vi "Counter with Button.vi"() -> ()   [LabVIEW 2022 SP3]
panel:
  in  "Sifirla":bool
  out "Say. Mavi":i32
  out "Say. Yesil":i32
  out "Say. Kirmizi":i32
  in  "stop":bool
  in  "Mavi":bool
  in  "Yesil":bool
  in  "Kirmizi":bool
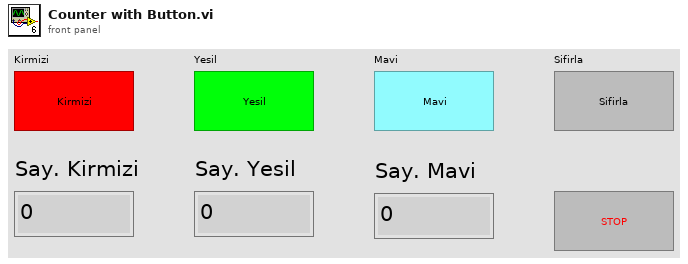
[diagram p1: front panel]
types:
  T1 = cluster{"Counters":cluster{"Say. Kirmizi":i32, "Say. Yesil":i32, "Say. Mavi":i32}}
  T2 = cluster{"Say. Kirmizi":i32, "Say. Yesil":i32, "Say. Mavi":i32}
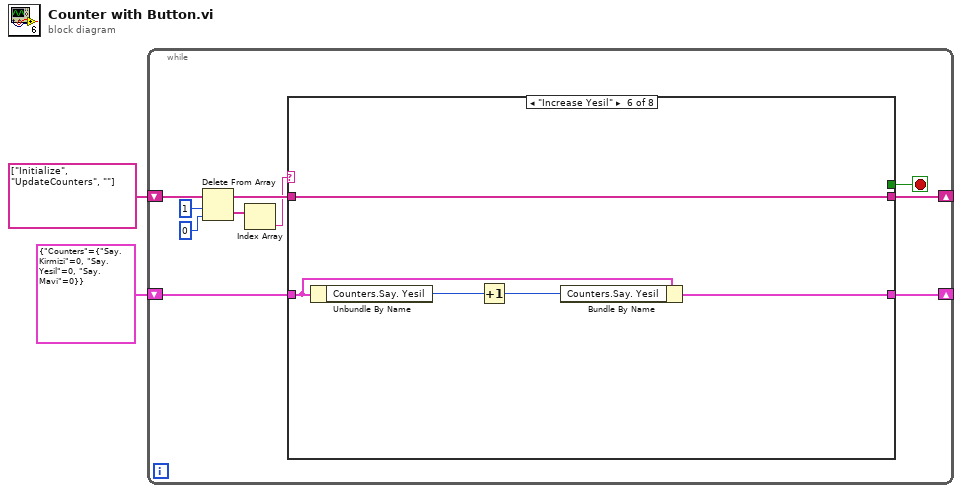
[diagram p0: block diagram]
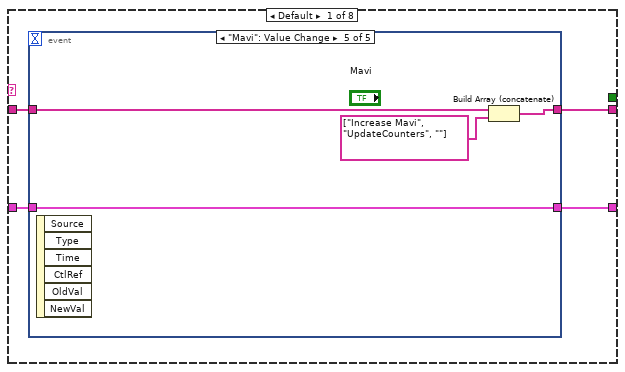
[diagram p2: hidden frame]
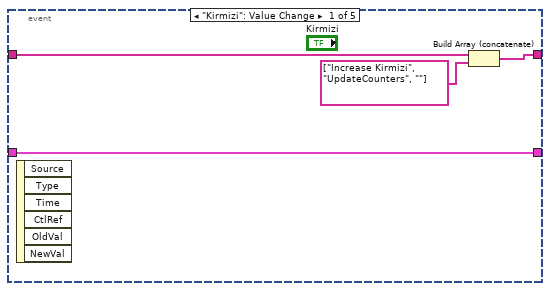
[diagram p3: hidden frame]
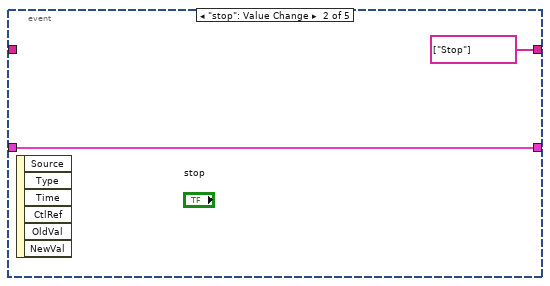
[diagram p4: hidden frame]
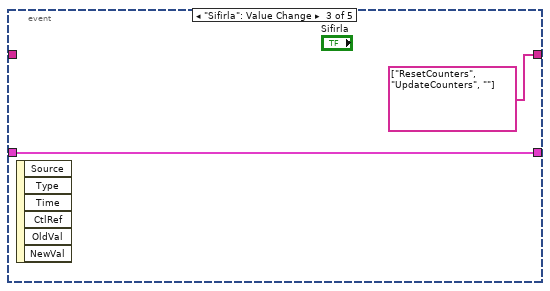
[diagram p5: hidden frame]
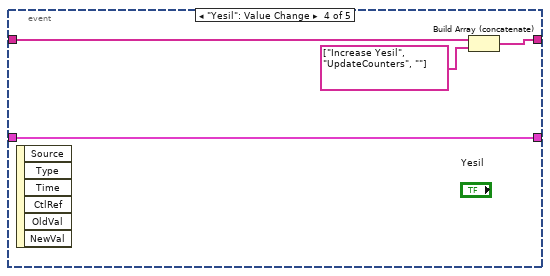
[diagram p6: hidden frame]
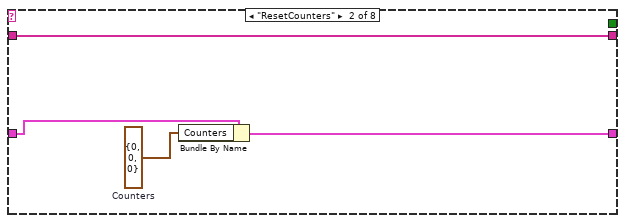
[diagram p7: hidden frame]
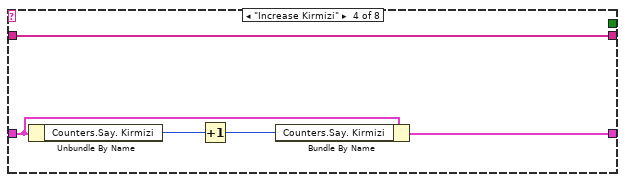
[diagram p9: hidden frame]
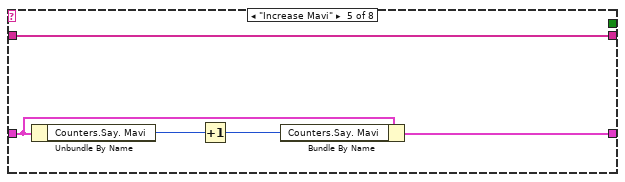
[diagram p10: hidden frame]
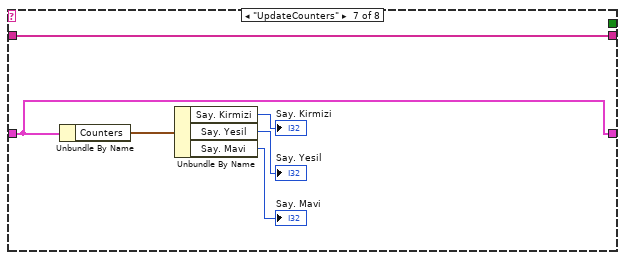
[diagram p11: hidden frame]
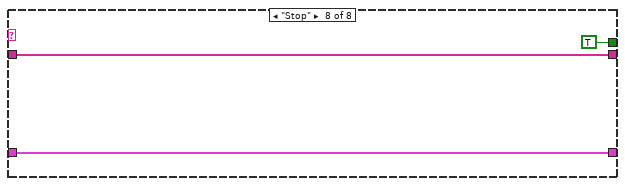
[diagram p12: hidden frame]
diagram:
  n1 = while {
    shift-right: [w10] -> _
    shift-left: T1 {"Counters"={"Say. Kirmizi"=0, "Say. Yesil"=0, "Say. Mavi"=0}} -> [w11]
    shift-right: [w3] -> _
    shift-left: string[] ["Initialize", "UpdateCounters", ""] -> [w9]
    stop <- w12 stop-if-true
    n2 = Delete From Array(array=w9, length=1, index=0) -> (deleted portion=w5:string[], array with subset deleted=w7:string[])
    n3 = Index Array(array=w5) -> (element=w4:string)  [unwired: 1 in]
    n4 = case shown="\"Increase Yesil\"" w4 {
      tunnel: [_ _ _ _ _ _ _ TRUE] -> w12
      tunnel: w11 -> [w16 w33 w38 w42 w47 w52 w58 w61]
      tunnel: [w15 w34 w38 w41 w46 w51 w58 w61] -> w10
      tunnel: w7 -> [w14 w36 w37 w43 w48 w53 w59 w60]
      tunnel: [w13 w36 w37 w43 w48 w53 w59 w60] -> w3
      frame Default {
        n5 = event shown="[4] \"Mavi\": Value Change" {
          selector: _ -> [_ _ _ _ _]
          dyn-events: _ -> [_ _ _ _ _]
          timeout: _ -> [_ _ _ _ _]
          tunnel: w16 -> [w20 w22 w24 w28 w32]
          tunnel: [w20 w22 w24 w28 w32] -> w15
          tunnel: w14 -> [w19 _ _ w27 w31]
          tunnel: [w18 string[] ["Stop"] string[] ["ResetCounters", "UpdateCounters", ""] w26 w30] -> w13
          event "Kirmizi": Value Change {
            n6 = event-data() -> ()  [unwired: 1 in, 6 out]
            n7 = Build Array (concatenate)(w19, string[] ["Increase Kirmizi", "UpdateCounters", ""]) -> (w18:string[])
          }
          event "stop": Value Change {
            n8 = event-data() -> ()  [unwired: 1 in, 6 out]
          }
          event "Sifirla": Value Change {
            n9 = event-data() -> ()  [unwired: 1 in, 6 out]
          }
          event "Yesil": Value Change {
            n10 = event-data() -> ()  [unwired: 1 in, 6 out]
            n11 = Build Array (concatenate)(w27, string[] ["Increase Yesil", "UpdateCounters", ""]) -> (w26:string[])
          }
          event "Mavi": Value Change {
            n12 = event-data() -> ()  [unwired: 1 in, 6 out]
            n13 = Build Array (concatenate)(w31, string[] ["Increase Mavi", "UpdateCounters", ""]) -> (w30:string[])
          }
        }
      }
      frame "ResetCounters" {
        w35 = T2 {"Say. Kirmizi"=0, "Say. Yesil"=0, "Say. Mavi"=0}  # Counters
        n14 = Bundle By Name(cluster=w33, "Counters"=w35) -> (w34:T1)
      }
      frame "Initialize" {
      }
      frame "Increase Kirmizi" {
        n15 = Unbundle By Name(w42) -> ("Counters.Say. Kirmizi"=w40:i32)
        n16 = Increment(x=w40) -> (x+1=w39:i32)
        n17 = Bundle By Name(cluster=w42, "Counters.Say. Kirmizi"=w39) -> (w41:T1)
      }
      frame "Increase Mavi" {
        n18 = Unbundle By Name(w47) -> ("Counters.Say. Mavi"=w45:i32)
        n19 = Increment(x=w45) -> (x+1=w44:i32)
        n20 = Bundle By Name(cluster=w47, "Counters.Say. Mavi"=w44) -> (w46:T1)
      }
      frame "Increase Yesil" {
        n21 = Unbundle By Name(w52) -> ("Counters.Say. Yesil"=w50:i32)
        n22 = Increment(x=w50) -> (x+1=w49:i32)
        n23 = Bundle By Name(cluster=w52, "Counters.Say. Yesil"=w49) -> (w51:T1)
      }
      frame "UpdateCounters" {
        n24 = Unbundle By Name(w58) -> ("Counters"=w57:T2)
        n25 = Unbundle By Name(w57) -> ("Say. Kirmizi"=→"Say. Kirmizi":i32, "Say. Yesil"=→"Say. Yesil":i32, "Say. Mavi"=→"Say. Mavi":i32)
      }
      frame "Stop" {
      }
    }
  }
